vi "Main.vi"() -> ()   [LabVIEW 2013]
doc: "Use this template to build a simple state machine design pattern. Each state executes code and determines which state to transition to."
uses:
  controls/Data.ctl
  <vilib>/express/express shared/transition.llb/Dynamic To Waveform Array.vi
  <vilib>/express/express shared/transition.llb/Waveform Array To Dynamic.vi
  <vilib>/express/express arith-compare/Formula/Block/exnFormulaBlock how many pts in the wave.vi
  <vilib>/express/express shared/ex_Modify Signal Name.vi
  <vilib>/express/express arith-compare/Formula/XNode/ExpressFormulaBlockNode.xnode
panel:
  out "Duty Cycle Graph":dynamicdata(graph)
  out "Coated Temperature graph":dynamicdata(graph)
  out "Bare temperature Graph":dynamicdata(graph)
  out "Elapsed time (sec)":dbl format="%#.3f"
  out "Rec count":dbl
  in  "Period (sec)":dbl=3.0
  out "Coated Temperature 2":dbl
  out "Bare Temperature 2":dbl
  out "Low Airflow":bool
  out "PWM On":bool
  out "PWM Graph":dynamicdata(graph)
  in  "Stop":bool=TRUE
  in  "Filename to save to":path=path "Z:/adit/Desktop/MEL III/RefrigerationData.lvm" caption="Filename"
  in  "Save Data?":bool=TRUE
  out "Derivative Output":dbl
  out "Integral Output":dbl
  out "CO Bias":dbl
  out "Proportional Output":dbl
  out "Duty Cycle":dbl
  out "Current Set Point":dbl
  out "Flow Rate":dbl
  in  "Integral Constant":dbl=0.1 caption="I Coefficient" format="%0.2f"
  in  "Derivative \nConstant":dbl=0.05 caption="D Coefficient" format="%0.2f"
  in  "Proportional\nConstant":dbl=1.0 caption="P Coefficient" format="%0.2f"
  in  "Duty Cycle\nincrement amount":dbl=1.0
  in  "Decrease Duty Cycle":bool
  in  "Increase Duty Cycle":bool
  in  "Set Point\nIncrement amount":dbl=1.0
  in  "Lower Set Point":bool
  in  "Raise Set Point":bool
  in  "Bare(T) or \nCoated?":bool
  in  "Manual / Auto":bool
  in  "Time to wait(ms)":u32
  in  "Readings between\nrecorded data":i32
  out "Bare Temperature":dbl
  out "Coated Temperature":dbl
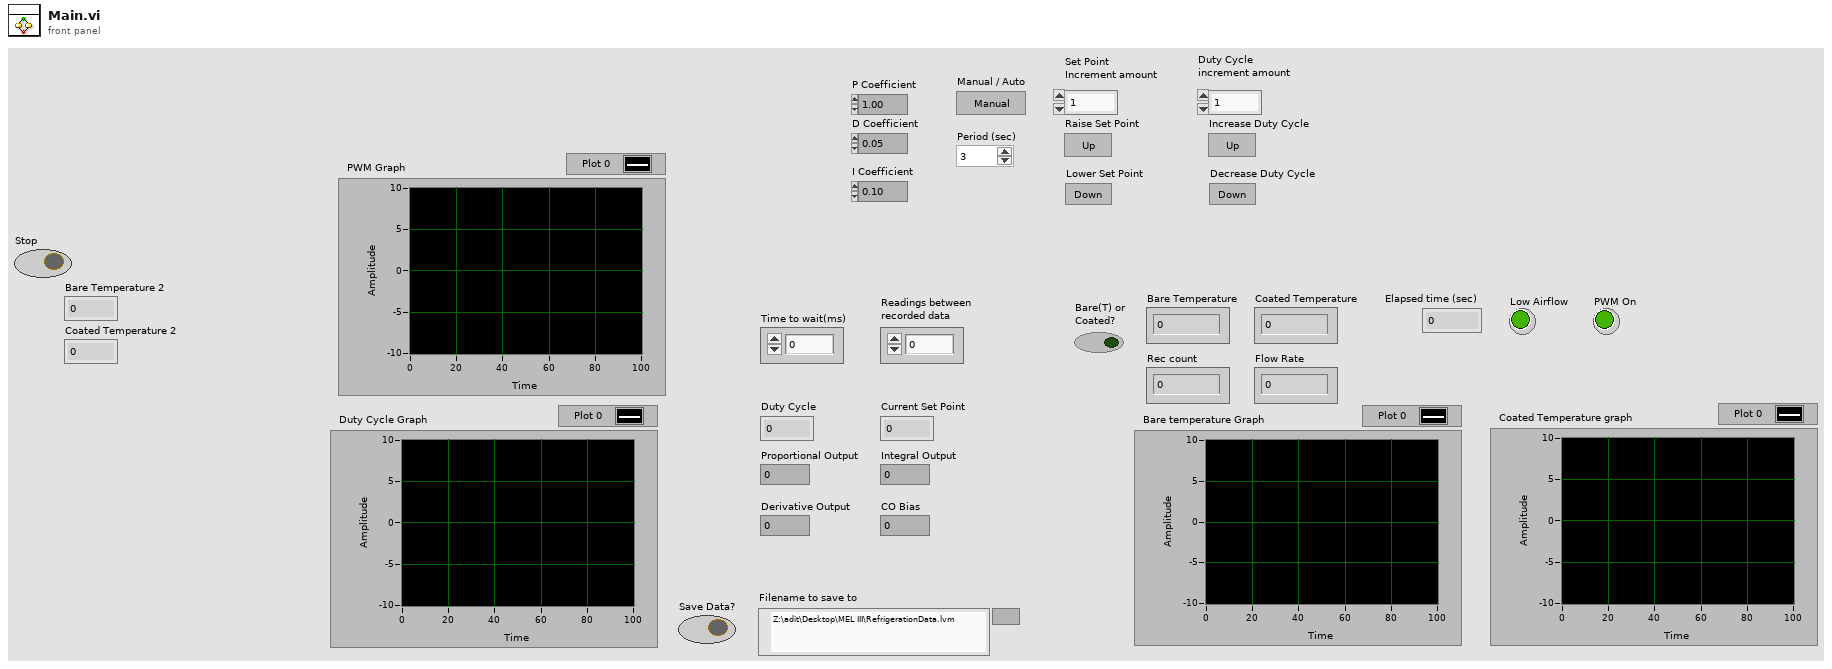
[diagram p1: front panel]
types:
  T1 = enum16{"Initialize", "Acquire", "Analyze", "PID", "Record", "PWM", "Output", ""}
  T2 = typedef "Data.ctl" = cluster{"Boolean <Replace Me>":bool, "String <Replace Me>":string, "Numeric <Replace Me>":dbl}
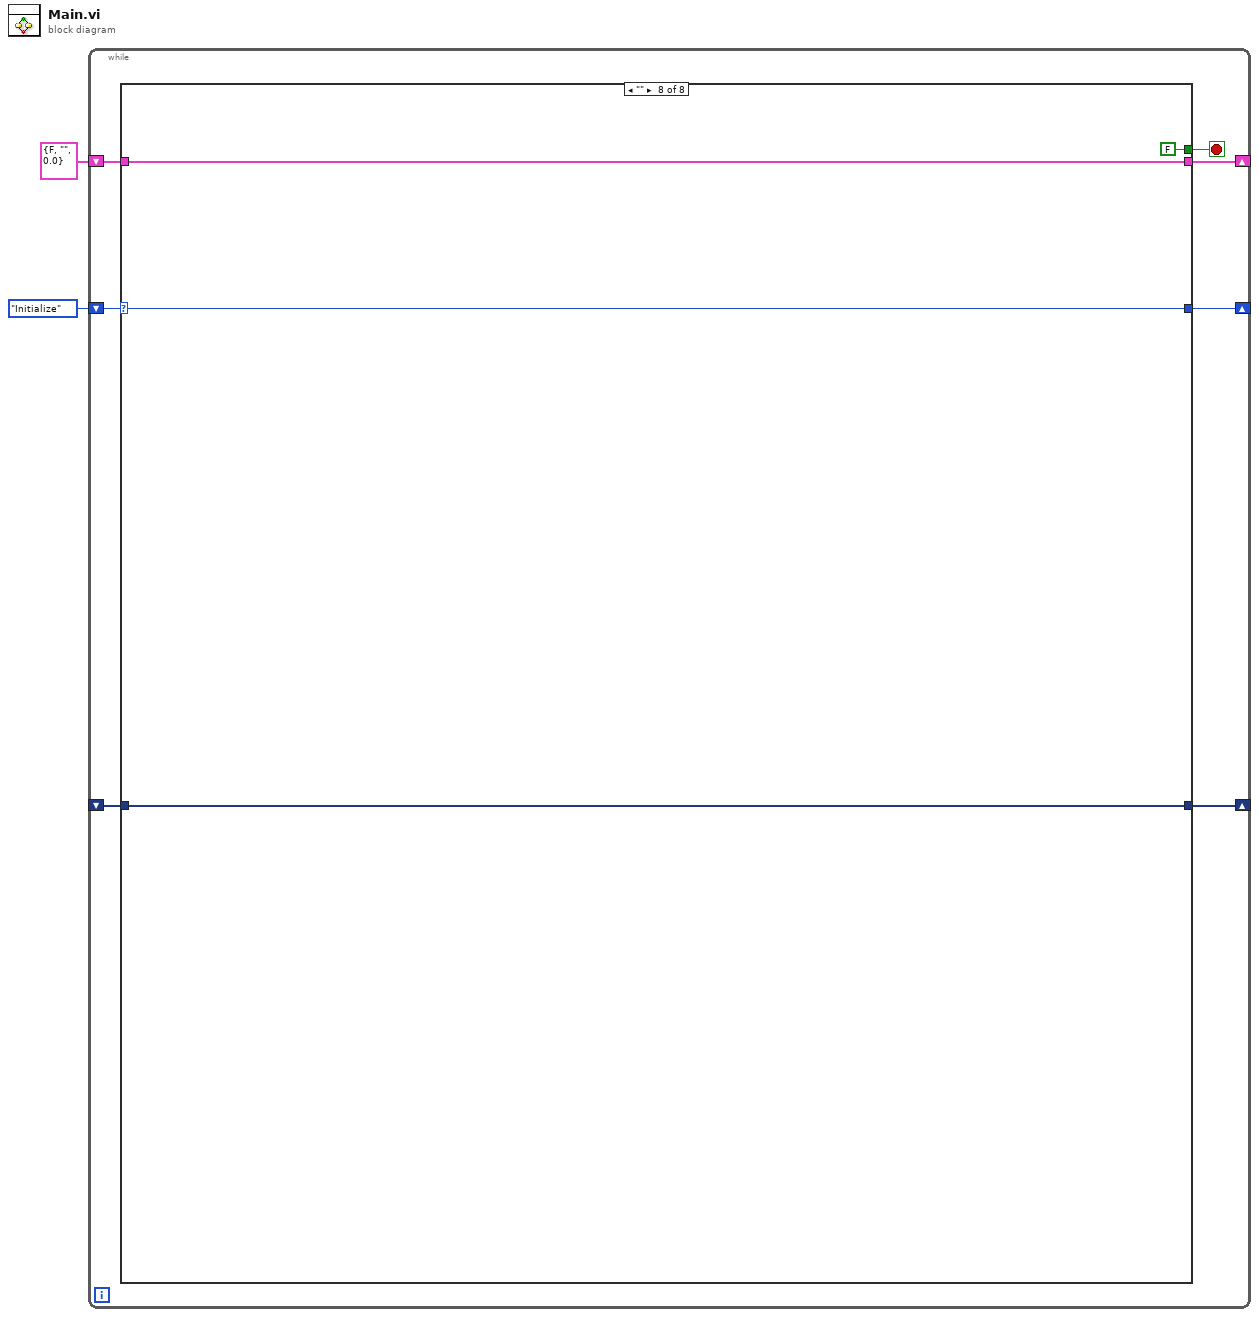
[diagram p0: block diagram]
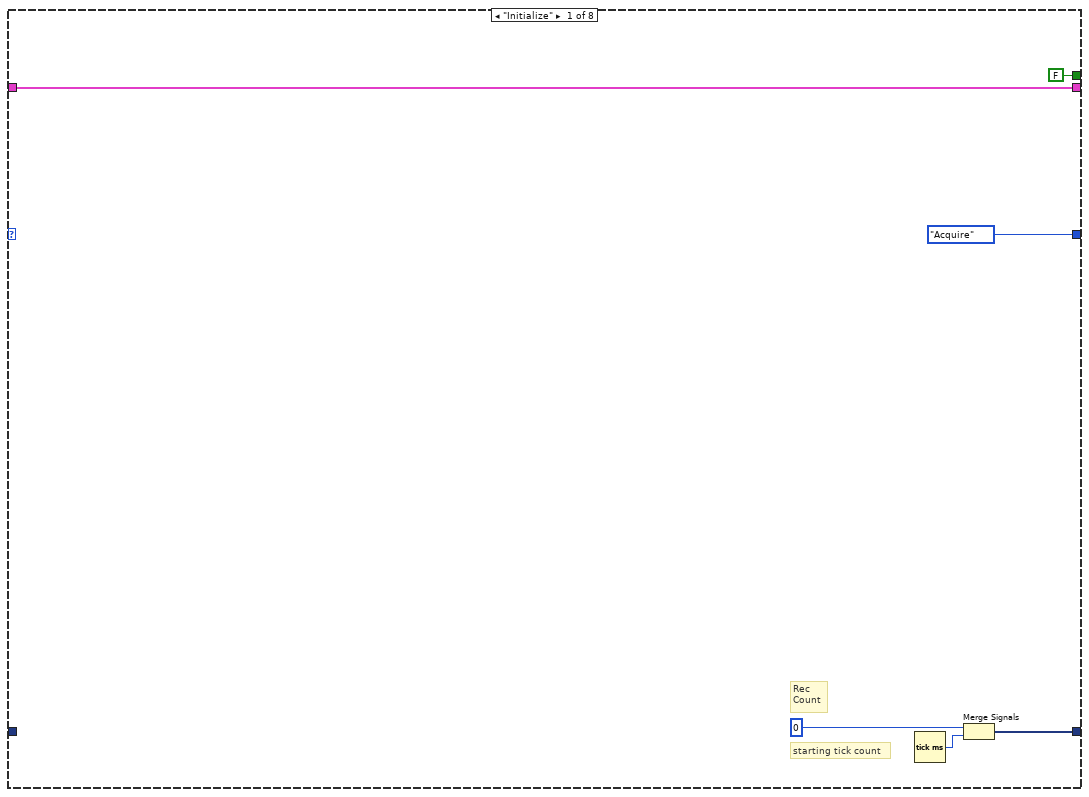
[diagram p2: hidden frame]
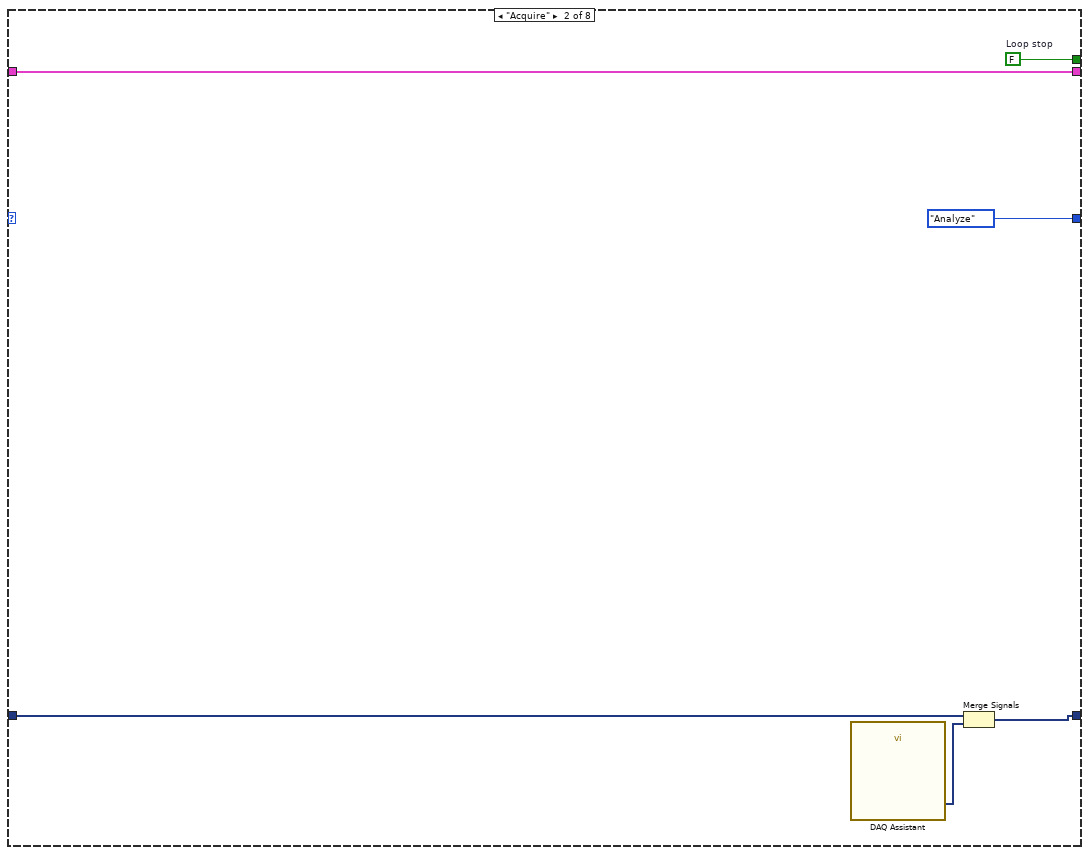
[diagram p3: hidden frame]
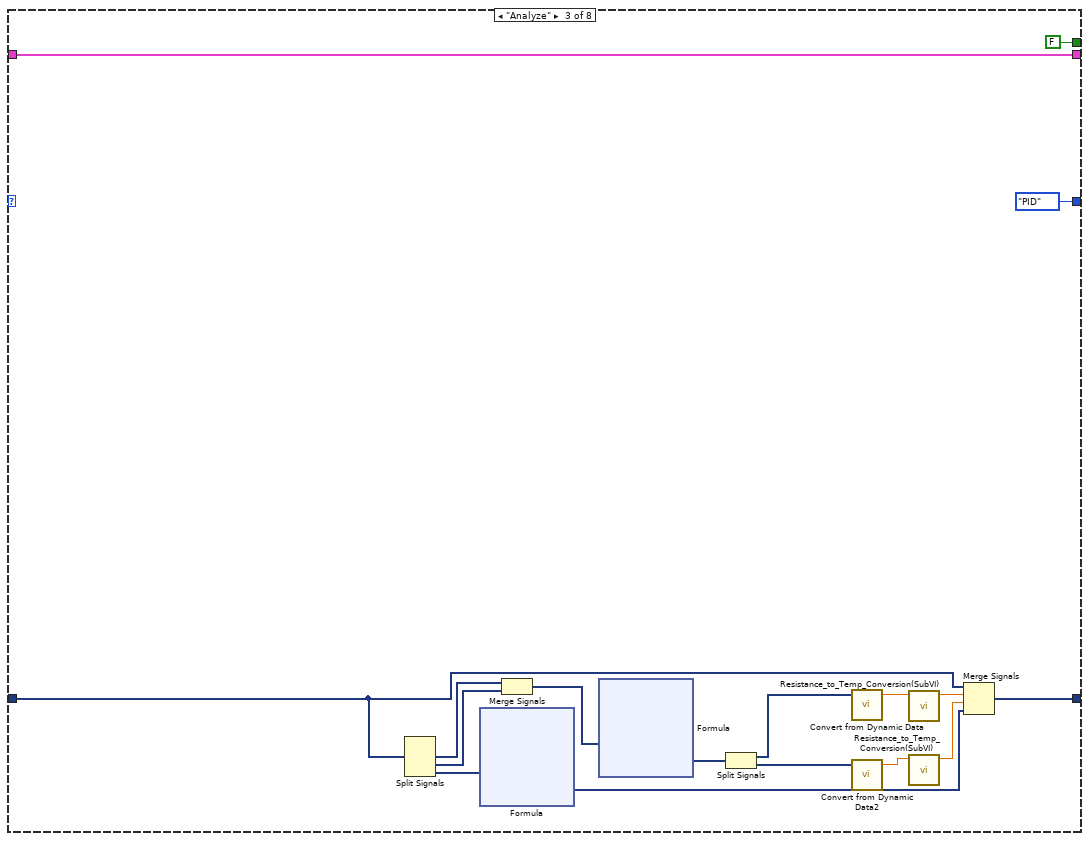
[diagram p4: hidden frame]
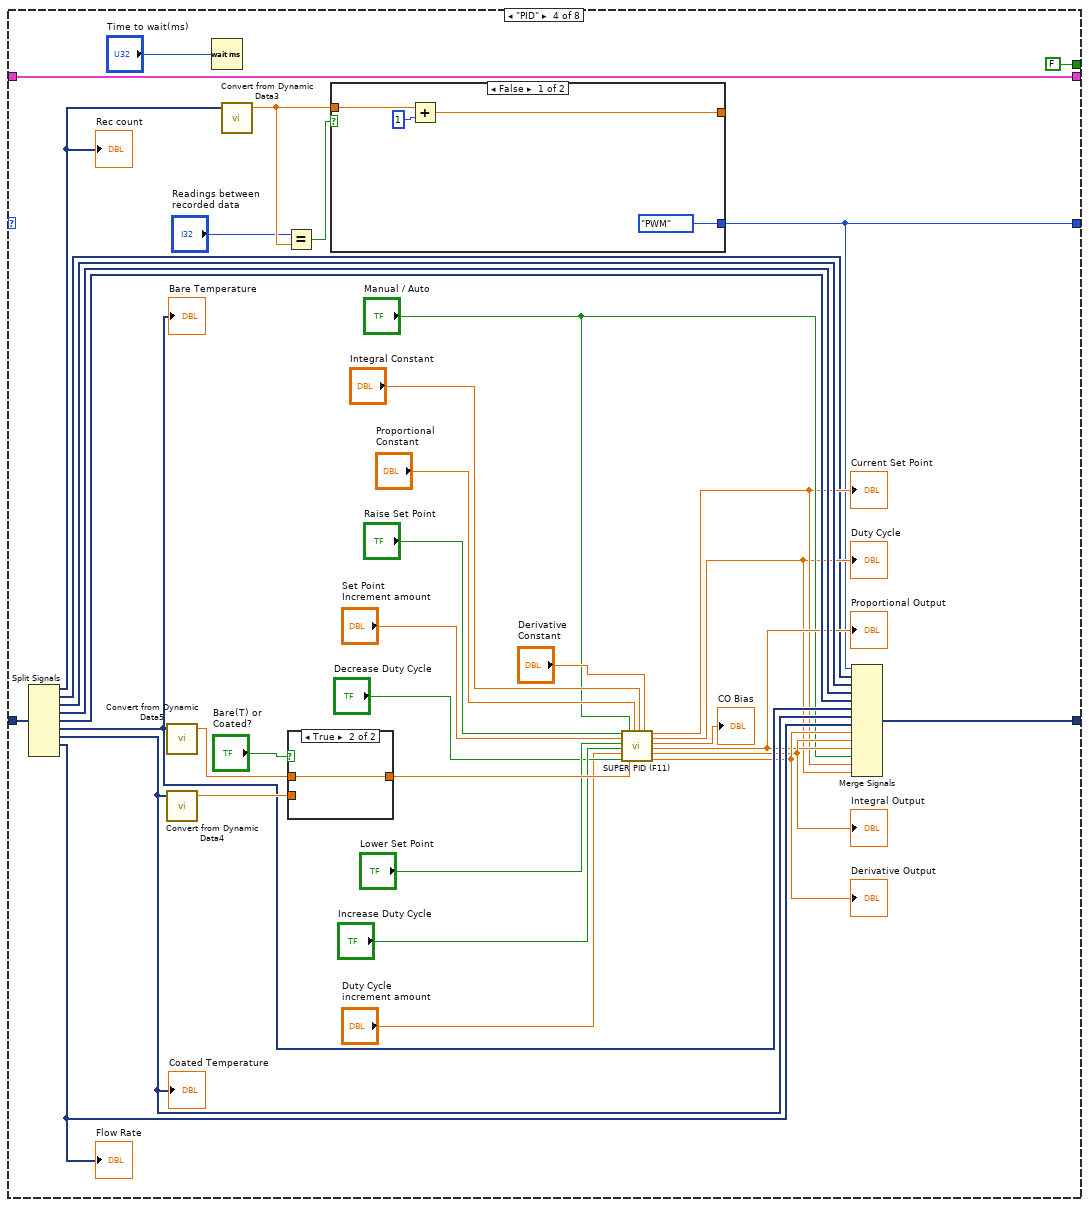
[diagram p5: hidden frame]
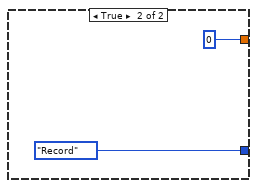
[diagram p7: hidden frame]
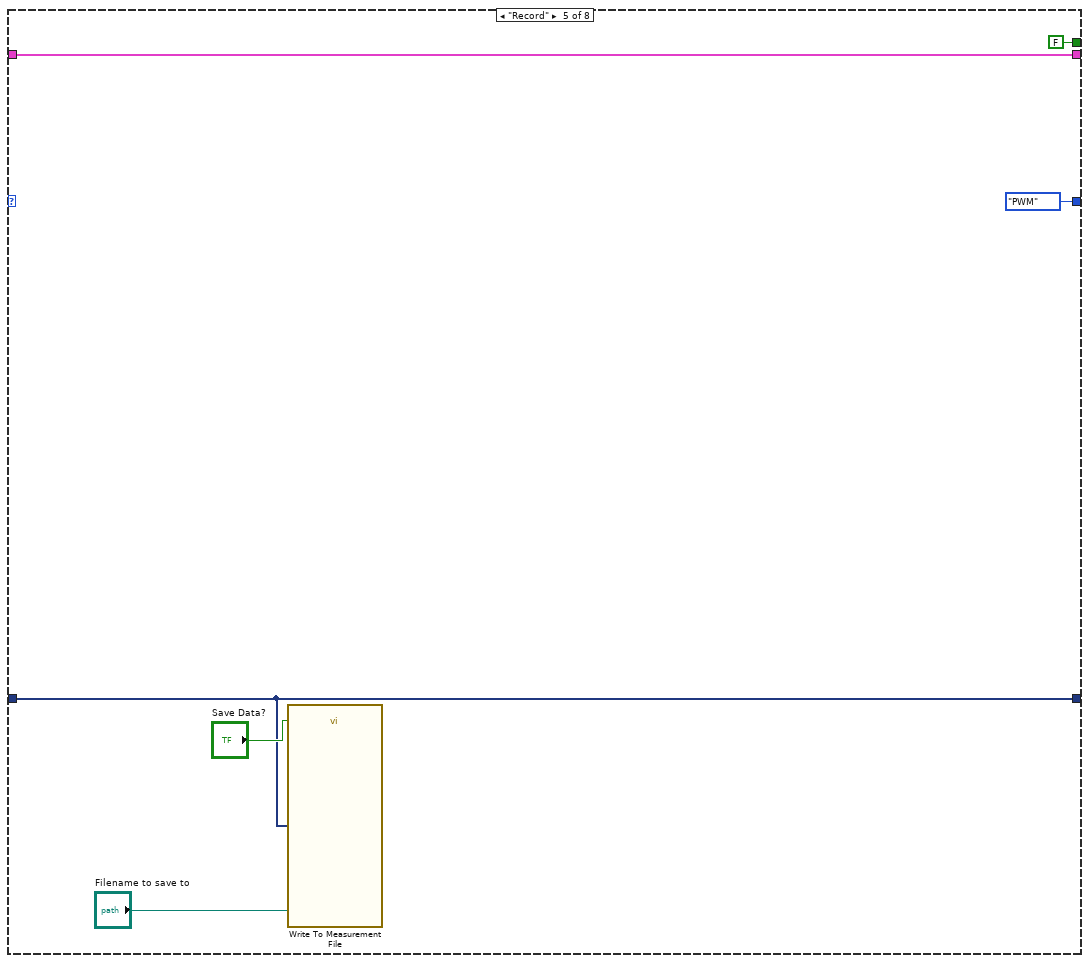
[diagram p8: hidden frame]
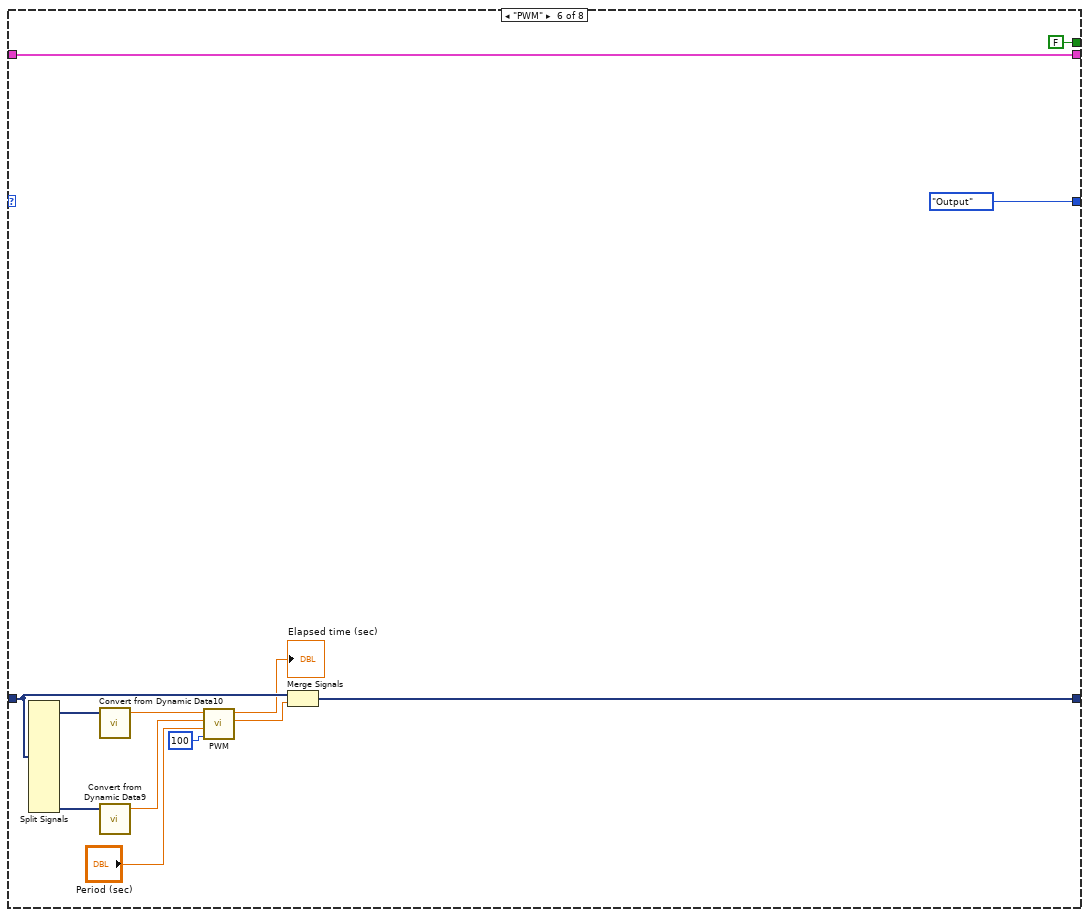
[diagram p9: hidden frame]
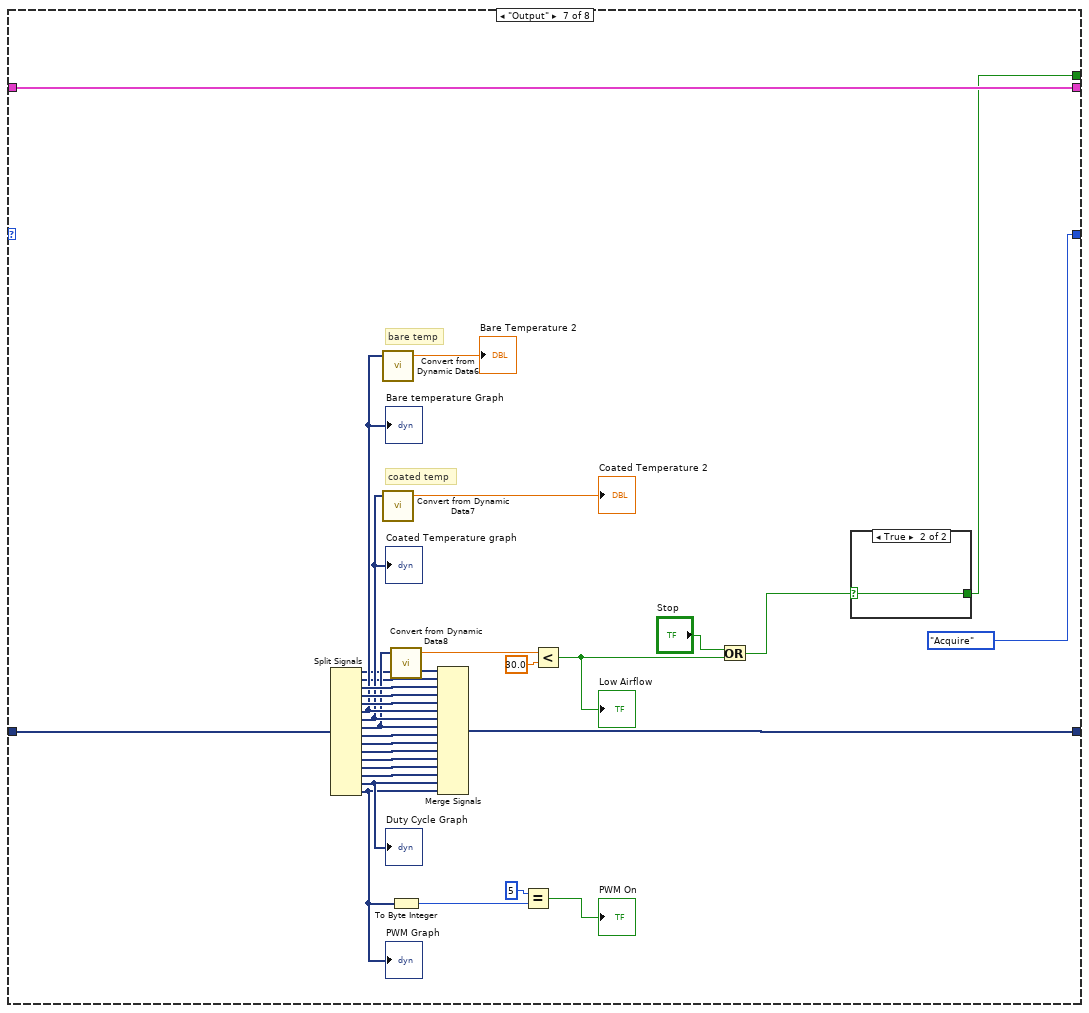
[diagram p10: hidden frame]
diagram:
  n1 = while {
    shift-right: [w8] -> _
    shift-left: T1."Initialize" -> [w9]
    shift-right: [w6] -> _
    shift-left: T2 {"Boolean <Replace Me>"=FALSE, "String <Replace Me>"="", "Numeric <Replace Me>"=0.0} ("Data") -> [w7]
    shift-right: [w4] -> _
    shift-left: _ -> [w3]
    stop <- w5 stop-if-true
    n2 = case shown="\"\"" w9 {
      selector: w9 -> [_ _ _ _ _ _ _ w415]
      tunnel: [T1."Acquire" T1."Analyze" T1."PID" w317 T1."PWM" T1."Output" T1."Acquire" w415] -> w8
      tunnel: [FALSE ("Stop Loop?") w21 FALSE ("Stop Loop?") FALSE ("Stop Loop?") FALSE ("Stop Loop?") FALSE ("Stop Loop?") w381 FALSE ("Stop Loop?")] -> w5
      tunnel: w7 -> [w11 w20 w37 w352 w367 w380 w411 w417]
      tunnel: [w11 w20 w37 w352 w367 w380 w411 w417] -> w6
      tunnel: [w12 w16 w22 w330 w363 w376 w387 w416] -> w4
      tunnel: w3 -> [_ w17 w23 w334 w363 w374 w386 w416]
      frame "Initialize" {
        # "starting tick count"
        # "Rec\nCount"
        n3 = Tick Count (ms)() -> (millisecond timer value=w13:u32)
        n4 = Merge Signals(0, w13) -> (w12:dynamicdata)
      }
      frame "Acquire" {
        w21 = FALSE  # Loop stop
        n5 = call "DAQ Assistant"() -> ("data"=w18:dynamicdata)  [unwired: 17 in, 2 out]
        n6 = Merge Signals(w17, w18) -> (w16:dynamicdata)
      }
      frame "Analyze" {
        n7 = Split Signals(w23) -> (w30:dynamicdata, w29:dynamicdata, w27:dynamicdata)  [unwired: 5 in, 2 out]
        n8 = xnode "Formula"("V"=w27) -> ("Result"=w26:dynamicdata)  [unwired: 1 in, 1 out]
        n9 = Merge Signals(w30, w29) -> (w28:dynamicdata)
        n10 = xnode "Formula"("V"=w28) -> ("Result"=w35:dynamicdata)  [unwired: 1 in, 1 out]
        n11 = Split Signals(w35) -> (w34:dynamicdata, w33:dynamicdata)  [unwired: 2 in]
        n12 = call "Convert from Dynamic Data"("Dynamic Data Type"=w34) -> ("Scalar"=w31:dbl)  [unwired: 3 in]
        n13 = call "Convert from Dynamic Data2"("Dynamic Data Type"=w33) -> ("Scalar"=w32:dbl)  [unwired: 3 in]
        n14 = call "Resistance_to_Temp_Conversion(SubVI).vi"("Scalar"=w31) -> ("Result"=w24:dbl)  [unwired: 10 in]
        n15 = call "Resistance_to_Temp_Conversion(SubVI).vi"("Scalar"=w32) -> ("Result"=w25:dbl)  [unwired: 10 in]
        n16 = Merge Signals(w23, w24, w25, w26) -> (w22:dynamicdata)
      }
      frame "PID" {
        n17 = Split Signals(w334) -> (w319:dynamicdata, w318:dynamicdata, w333:dynamicdata, w332:dynamicdata, w331:dynamicdata, w327:dynamicdata, w326:dynamicdata, w328:dynamicdata)  [unwired: 9 in, 1 out]
        "Coated Temperature" <- w326
        "Bare Temperature" <- w327
        "Flow Rate" <- w328
        "Rec count" <- w319
        n18 = call "Convert from Dynamic Data5"("Dynamic Data Type"=w327) -> ("Scalar"=w347:dbl)  [unwired: 3 in]
        n19 = call "Convert from Dynamic Data4"("Dynamic Data Type"=w326) -> ("Scalar"=w348:dbl)  [unwired: 3 in]
        n20 = Wait (ms)(milliseconds to wait="Time to wait(ms)") -> ()  [unwired: 1 out]
        n21 = call "Convert from Dynamic Data3"("Dynamic Data Type"=w319) -> ("Scalar"=w351:dbl)  [unwired: 3 in]
        n22 = Equal?(x="Readings between\nrecorded data", y=w351) -> (x = y?=w335:bool)
        n23 = case shown="True" "Bare(T) or \nCoated?" {
          tunnel: w348 -> [w354 _]
          tunnel: w347 -> [_ w355]
          tunnel: [w354 w355] -> w346
          frame False {
          }
          frame True {
          }
        }
        n24 = case shown="False" w335 {
          tunnel: [T1."PWM" T1."Record"] -> w317
          tunnel: w351 -> [w358 _]
          tunnel: [w356 0] -> _
          frame False {
            n25 = Add(x=w358, y=1) -> (x+y=w356:dbl)
          }
          frame True {
          }
        }
        n26 = call "SUPER PID (F11).vi"("SP Up"="Raise Set Point", "SP Increment"="Set Point\nIncrement amount", "SP Down"="Lower Set Point", "DC Up"="Increase Duty Cycle", "DC Increment"="Duty Cycle\nincrement amount", "DC Down"="Decrease Duty Cycle", "Manual / Auto"="Manual / Auto", "PV"=w346, "P"="Proportional\nConstant", "I"="Integral Constant", "D"="Derivative \nConstant") -> ("SP"=w321:dbl, "DC"=w320:dbl, "CO Bias"=→"CO Bias":dbl, "P out"=w323:dbl, "I out"=w324:dbl, "D out"=w325:dbl)  [unwired: 3 in]
        "Current Set Point" <- w321
        "Duty Cycle" <- w320
        "Proportional Output" <- w323
        "Integral Output" <- w324
        "Derivative Output" <- w325
        n27 = Merge Signals(w317, w318, w333, w332, w331, w327, w326, w328, w325, w324, w323, "Manual / Auto", w321, w320) -> (w330:dynamicdata)
      }
      frame "Record" {
        n28 = call "Write To Measurement File"("Signals"=w363, "Reset"="Save Data?", "Filename"="Filename to save to") -> ()  [unwired: 14 in, 3 out]
      }
      frame "PWM" {
        n29 = Split Signals(w374) -> (w373:dynamicdata, w370:dynamicdata)  [unwired: 14 in, 12 out]
        n30 = call "Convert from Dynamic Data10"("Dynamic Data Type"=w373) -> ("Scalar"=w372:dbl)  [unwired: 3 in]
        n31 = call "Convert from Dynamic Data9"("Dynamic Data Type"=w370) -> ("Scalar"=w371:dbl)  [unwired: 3 in]
        n32 = call "PWM.vi"("milliseconds to wait"=u32 100, "Period (sec)"="Period (sec)", "Duty Cycle"=w371, "Starting tic count"=w372) -> ("Pwm output"=w377:dbl, "Elapsed time (sec)"=→"Elapsed time (sec)":dbl)  [unwired: 6 in]
        n33 = Merge Signals(w374, w377) -> (w376:dynamicdata)
      }
      frame "Output" {
        # "coated temp"
        # "bare temp"
        n34 = Split Signals(w386) -> (w383:dynamicdata, w384:dynamicdata, w399:dynamicdata, w398:dynamicdata, w397:dynamicdata, w396:dynamicdata, w395:dynamicdata, w394:dynamicdata, w393:dynamicdata, w392:dynamicdata, w391:dynamicdata, w390:dynamicdata, w389:dynamicdata, w388:dynamicdata, w385:dynamicdata, w382:dynamicdata)  [unwired: 16 in]
        "PWM Graph" <- w382
        "Bare temperature Graph" <- w396
        "Coated Temperature graph" <- w395
        "Duty Cycle Graph" <- w385
        n35 = call "Convert from Dynamic Data6"("Dynamic Data Type"=w396) -> ("Scalar"=→"Bare Temperature 2":dbl)  [unwired: 3 in]
        n36 = call "Convert from Dynamic Data7"("Dynamic Data Type"=w395) -> ("Scalar"=→"Coated Temperature 2":dbl)  [unwired: 3 in]
        n37 = call "Convert from Dynamic Data8"("Dynamic Data Type"=w394) -> ("Scalar"=w404:dbl)  [unwired: 3 in]
        n38 = To Byte Integer(number=w382) -> (8bit integer=w408:i8)
        n39 = Merge Signals(w383, w384, w399, w398, w397, w396, w395, w394, w393, w392, w391, w390, w389, w388, w385, w382) -> (w387:dynamicdata)
        n40 = Equal?(x=5, y=w408) -> (x = y?=→"PWM On":bool)
        n41 = Less?(x=w404, y=30.0) -> (x < y?=w403:bool)
        "Low Airflow" <- w403
        n42 = Or(x="Stop", y=w403) -> (x .or. y?=w400:bool)
        n43 = case shown="True" w400 {
          selector: w400 -> [w412 w413]
          tunnel: [w412 w413] -> w381
          frame False {
          }
          frame True {
          }
        }
      }
      frame "" {
      }
    }
  }
